vi "CN Switch Page.vi"(3 "Page":i32, 4 "Scond":dbl=10.0 format="%#_13g", 5 "Tab":T1(array[ring])) -> (0 "x >= y?":bool, 1 "Page":i32, 2 "scond":dbl)   [LabVIEW 2014]
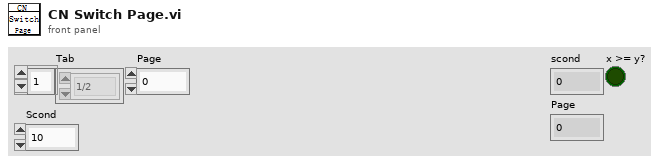
[diagram p1: front panel]
types:
  T1 = enum32{"1/2", "1/3", "1/4", "1/5", "2/5", "3/5"}[]
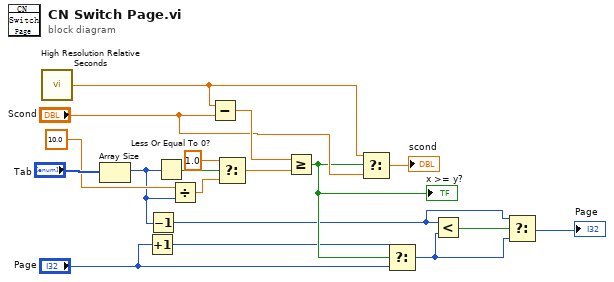
[diagram p0: block diagram]
diagram:
  n1 = call <vilib>:"High Resolution Relative Seconds.vi"() -> ("relative seconds"=w11:dbl)
  n2 = Array Size(array="Tab") -> (size(s)=w5:i32)
  n3 = Increment(x="Page") -> (x+1=w6:i32)
  n4 = Decrement(x=w5) -> (x-1=w3:i32)
  n5 = Less Or Equal To 0?(x=w5) -> (x <= 0?=w17:bool)
  n6 = Divide(x=10.0, y=w5) -> (x/y=w15:dbl)
  n7 = Subtract(x=w11, y="Scond") -> (x-y=w12:dbl)
  n8 = Select(t=1.0, s=w17, f=w15) -> (s? t:f=w13:dbl)
  n9 = Greater Or Equal?(x=w12, y=w13) -> (x >= y?=w8:bool)
  "x >= y?" <- w8
  n10 = Select(t=w11, s=w8, f="Scond") -> (s? t:f=→"scond":dbl)
  n11 = Select(t=w6, s=w8, f="Page") -> (s? t:f=w1:i32)
  n12 = Less?(x=w3, y=w1) -> (x < y?=w4:bool)
  n13 = Select(t=w3, s=w4, f=w1) -> (s? t:f=→"Page":i32)
